vi "Poles_Placement.vi"(8 "Desired Poles":cdb[](array[numeric]) format="%#.6g", 11 "State-Space Model":T1 {"Transport Delay" format="%.2f"; "D" format="%#.2g"; "C" format="%#.2g"; "B" format="%#.2g"; "A" format="%#.2g"; "properties"."Sampling Time" format="%#.6p"; "properties"."Output Delays" format="%.4f"; "properties"."Input Delays" format="%.4f"}) -> (0 "Gain 2":dbl[][](array[numeric]) format="%.2f", 1 "Gain":dbl[](array[numeric]), 2 "State Trajectory Graph":cluster{"time":dbl[], dbl[]}[](graph), 3 "Closed-Loop Step Response":cluster{"time":dbl[], dbl[]}[](graph), 4 "Actual Poles":cdb[](array[numeric])=[-4.9512521676495505+0.0i, -3.4076115316471447-10.013861291935113i, -3.4076115316471447+10.013861291935113i] format="%.2f", 5 "Desired Poles":cdb[](array[numeric])=[-4.951252167649562+0.0i, -3.4076115316471642-10.013861291935129i, -3.4076115316471642+10.013861291935129i] format="%.2f")   [LabVIEW 2017]
uses:
  <vilib>/addons/Control Design/_Model Construction/Model Typedefs.llb/CD State Space Model (MIMO).ctl
  <vilib>/addons/Control Design/_Model Construction/Model Typedefs.llb/CD General Elements.ctl
  <vilib>/addons/Control Design/_Model Construction/Data Typedefs.llb/CD Time Info.ctl
  <vilib>/Analysis/polynomials.llb/Sort Complex Numbers (obs).vi
  <vilib>/addons/Control Design/_State Feedback Control/State Feedback Control.llb/CD State Regulator.vi
  <vilib>/addons/Control Design/_Time Response Analysis/Time Response.llb/Time Response subVI/cd_Step Response (State-Space).vi
  <vilib>/Analysis/NI_AALPro.lvlib
  <vilib>/addons/Control Design/_Model Construction/NI_LinSys_Data Typedefs.lvlib
  <vilib>/addons/Control Design/_Time Response Analysis/NI_CD_Time Response.lvlib
  <vilib>/addons/Control Design/_State Feedback Control/NI_CD_State Feedback Control.lvlib
  <vilib>/addons/Control Design/_Model Construction/NI_LinSys_Model Typedefs.lvlib
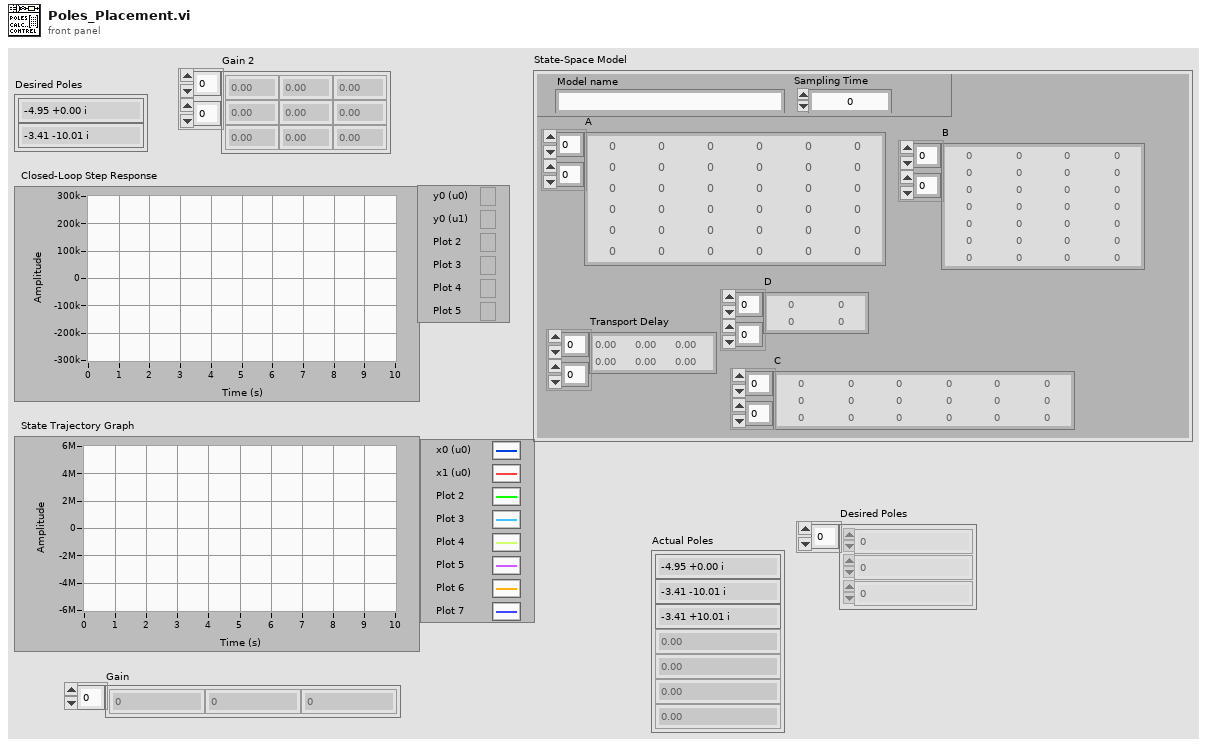
[diagram p1: front panel]
types:
  T1 = typedef "NI_LinSys_Model Typedefs.lvlib/CD State Space Model (MIMO).ctl" = cluster{"properties":T2, "A":dbl[][], "B":dbl[][], "C":dbl[][], "D":dbl[][], "StateNames":string[], "Transport Delay":dbl[][]}
  T2 = typedef "NI_LinSys_Model Typedefs.lvlib/CD General Elements.ctl" = cluster{"Model name":string, "Input names":string[], "Output names":string[], "Input Delays":dbl[], "Output Delays":dbl[], "Sampling Time":dbl, "Notes":string}
  T3 = typedef "NI_LinSys_Data Typedefs.lvlib/CD Time Info.ctl" = cluster{"t0":dbl, "dt":dbl, "tf":dbl}
  T4 = enum16{"System Included", "System Included with Noise", "Standalone"}
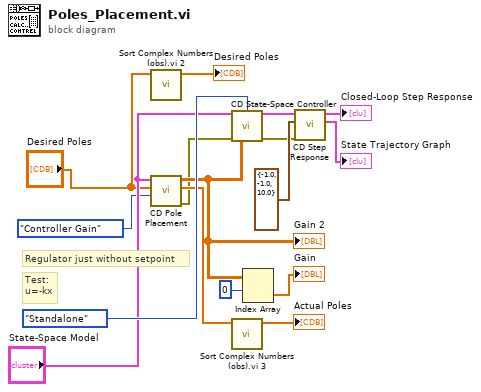
[diagram p0: block diagram]
diagram:
  # "Test:\nu=-kx"
  # "Regulator just without setpoint"
  n1 = call "Sort Complex Numbers (obs).vi 2"("Complex Numbers"="Desired Poles") -> ("Sorted Complex Numbers"=→"Desired Poles":cdb[])  [unwired: 8 in, 2 out]
  n2 = call <vilib>:"CD Pole Placement.vi"("Gain Type"=enum16{"Controller Gain", "Observer Gain"}."Controller Gain" ("Type"), "Poles"="Desired Poles", "State-Space Model"="State-Space Model") -> ("error out"=w2:errorcluster, "Actual Poles"=w7:cdb[], "Gain"=w6:dbl[][])  [unwired: 6 in]
  "Gain 2" <- w6
  n3 = call-poly <vilib>:"CD State-Space Controller.vi"("State-Space Model"="State-Space Model", "Configuration"=T4."Standalone", "error in (no error)"=w2, "Controller Gain (K)"=w6) -> ("Controller Model"=w12:T1, "error out"=w1:errorcluster)  [unwired: 10 in]
  n4 = call "Sort Complex Numbers (obs).vi 3"("Complex Numbers"=w7) -> ("Sorted Complex Numbers"=→"Actual Poles":cdb[])  [unwired: 8 in, 2 out]
  n5 = Index Array(array=w6, index (row)=0) -> (element=→"Gain":dbl[])  [unwired: 1 in]
  n6 = call-poly <vilib>:"CD Step Response.vi"("error in (no error)"=w1, "Time Range"=T3 {"t0"=-1.0, "dt"=-1.0, "tf"=10.0} ("Time Info"), "State-Space Model"=w12) -> ("State Trajectory Graph"=→"State Trajectory Graph":cluster{"time":dbl[], dbl[]}[], "Step Response Graph"=→"Closed-Loop Step Response":cluster{"time":dbl[], dbl[]}[])  [unwired: 5 in, 2 out]
